vi "IVIS FRET_Compute Ratios.vi"(9 "g":dbl=1.0 min=0.0, 11 "Frame Image Components":T3) -> (1 "Frame Image Parameters":T2, 2 "Frame Image Intensities":T1, 3 "Frame Image Outputs":T5)   [LabVIEW 2021]
uses:
  IVIS FRET_Frame Image Outputs.ctl
  IVIS FRET_Frame Image Components Data.ctl
  Image/Image Point.ctl
  IVIS FRET_Frame Image Parameters.ctl
  IVIS FRET_Frame Image Intensities.ctl
  b41ef2ff-39d0-4c19-96d8-b3aa1b28ecf1.vi
  7645d199-fdb0-4455-8b8c-9fcb5e39c3d7.vi
  9ac8a814-4e7f-4100-867f-6759366377cb.vi
  41b5a819-f782-48c6-95c8-fb2ee3cdc111.vi
  b41ef2ff-39d0-4c19-96d8-b3aa1b28ecf1.vi/1ce800e1-bcd7-4855-83e2-66cab3687e54.vi
  7645d199-fdb0-4455-8b8c-9fcb5e39c3d7.vi/1ce800e1-bcd7-4855-83e2-66cab3687e54.vi
  9ac8a814-4e7f-4100-867f-6759366377cb.vi/1ce800e1-bcd7-4855-83e2-66cab3687e54.vi
  41b5a819-f782-48c6-95c8-fb2ee3cdc111.vi/1ce800e1-bcd7-4855-83e2-66cab3687e54.vi
  <vilib>/Analysis/NI_AALBase.lvlib
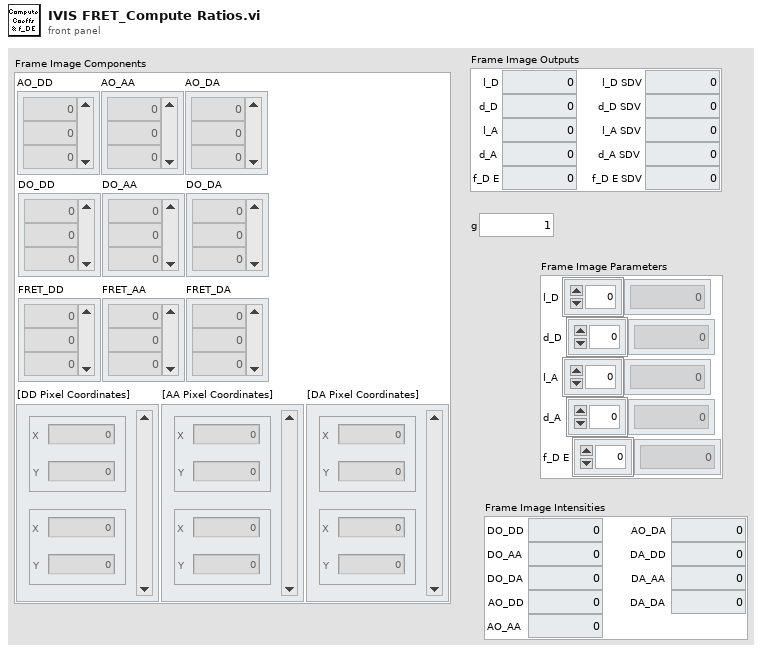
[diagram p1: front panel]
types:
  T1 = typedef "IVIS FRET_Frame Image Intensities.ctl" = cluster{"DO_DD":dbl, "DO_AA":dbl, "DO_DA":dbl, "AO_DD":dbl, "AO_AA":dbl, "AO_DA":dbl, "DA_DD":dbl, "DA_AA":dbl, "DA_DA":dbl}
  T2 = typedef "IVIS FRET_Frame Image Parameters.ctl" = cluster{"l_D":dbl[], "d_D":dbl[], "l_A":dbl[], "d_A":dbl[], "f_D E":dbl[]}
  T3 = typedef "IVIS FRET_Frame Image Components Data.ctl" = cluster{"AO_DD":sgl[], "AO_AA":sgl[], "AO_DA":sgl[], "DO_DA":sgl[], "DO_AA":sgl[], "DO_DD":sgl[], "FRET_DA":sgl[], "FRET_AA":sgl[], "FRET_DD":sgl[], "[DD Pixel Coordinates]":T4[], "[AA Pixel Coordinates]":T4[], "[DA Pixel Coordinates]":T4[]}
  T4 = typedef "Image Point.ctl" = cluster{"X":i32, "Y":i32}
  T5 = typedef "IVIS FRET_Frame Image Outputs.ctl" = cluster{"l_D":dbl, "l_D SDV":dbl, "d_D":dbl, "d_D SDV":dbl, "l_A":dbl, "l_A SDV":dbl, "d_A":dbl, "d_A SDV":dbl, "f_D E":dbl, "f_D E SDV":dbl}
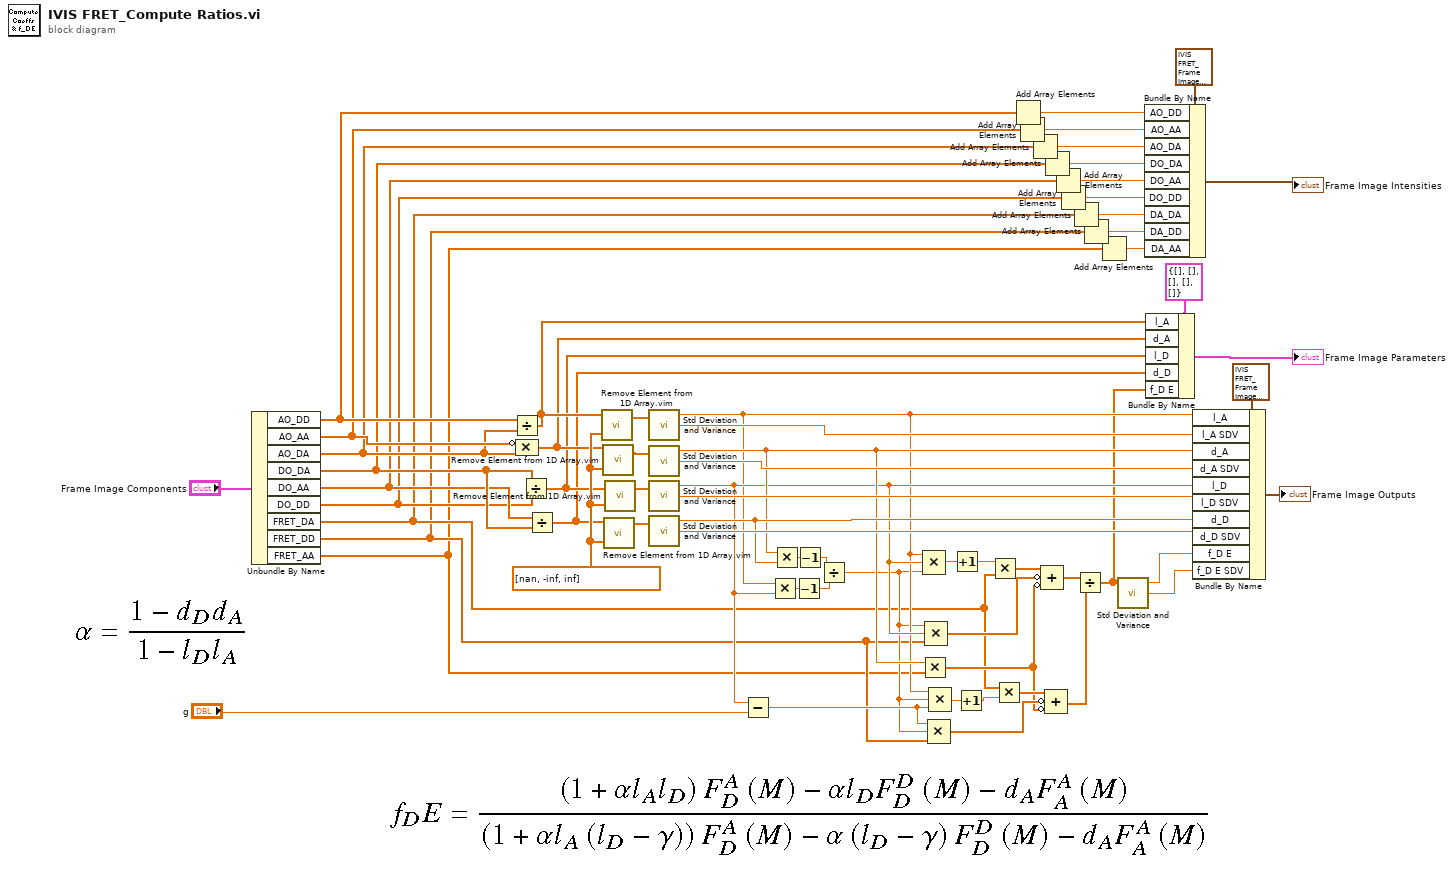
[diagram p0: block diagram]
diagram:
  w28 = dbl[] [nan, -inf, inf] ("Element(s) to Remove")
  n1 = Unbundle By Name("Frame Image Components") -> ("AO_DD"=w18:sgl[], "AO_AA"=w17:sgl[], "AO_DA"=w16:sgl[], "DO_DA"=w15:sgl[], "DO_AA"=w14:sgl[], "DO_DD"=w13:sgl[], "FRET_DA"=w12:sgl[], "FRET_DD"=w11:sgl[], "FRET_AA"=w10:sgl[])
  n2 = Divide(x=w18, y=w16) -> (x/y=w25:sgl[])
  n3 = Compound Arithmetic op=MULTIPLY(invert w17, w16) -> (w24:sgl[])
  n4 = Divide(x=w15, y=w13) -> (x/y=w23:sgl[])
  n5 = Divide(x=w14, y=w15) -> (x/y=w22:sgl[])
  n6 = call "Remove Element from 1D Array.vim"("Element(s) to Remove"=w28, "Input Array"=w25) -> ("Output Array"=w32:sgl[])  [unwired: 1 out]
  n7 = call "Remove Element from 1D Array.vim"("Element(s) to Remove"=w28, "Input Array"=w24) -> ("Output Array"=w29:sgl[])  [unwired: 1 out]
  n8 = call "Remove Element from 1D Array.vim"("Element(s) to Remove"=w28, "Input Array"=w22) -> ("Output Array"=w30:sgl[])  [unwired: 1 out]
  n9 = call "Remove Element from 1D Array.vim"("Element(s) to Remove"=w28, "Input Array"=w23) -> ("Output Array"=w31:sgl[])  [unwired: 1 out]
  n10 = call <vilib>:"Std Deviation and Variance.vi"("X"=w32) -> ("mean"=w44:dbl, "standard deviation"=w59:dbl)  [unwired: 1 in, 1 out]
  n11 = call <vilib>:"Std Deviation and Variance.vi"("X"=w29) -> ("mean"=w47:dbl, "standard deviation"=w57:dbl)  [unwired: 1 in, 1 out]
  n12 = call <vilib>:"Std Deviation and Variance.vi"("X"=w31) -> ("mean"=w46:dbl, "standard deviation"=w61:dbl)  [unwired: 1 in, 1 out]
  n13 = call <vilib>:"Std Deviation and Variance.vi"("X"=w30) -> ("mean"=w56:dbl, "standard deviation"=w58:dbl)  [unwired: 1 in, 1 out]
  n14 = Subtract(x=w46, y="g") -> (x-y=w40:dbl)
  n15 = Multiply(x=w44, y=w46) -> (x*y=w54:dbl)
  n16 = Multiply(x=w47, y=w56) -> (x*y=w55:dbl)
  n17 = Decrement(x=w54) -> (x-1=w52:dbl)
  n18 = Decrement(x=w55) -> (x-1=w53:dbl)
  n19 = Divide(x=w53, y=w52) -> (x/y=w39:dbl)
  n20 = Multiply(x=w47, y=w10) -> (x*y=w37:dbl[])
  n21 = Compound Arithmetic op=MULTIPLY(w44, w46, w39) -> (w51:dbl)
  n22 = Compound Arithmetic op=MULTIPLY(w39, w46, w11) -> (w48:dbl[])
  n23 = Compound Arithmetic op=MULTIPLY(w40, w39, w11) -> (w38:dbl[])
  n24 = Compound Arithmetic op=MULTIPLY(w44, w39, w40) -> (w43:dbl)
  n25 = Increment(x=w51) -> (x+1=w50:dbl)
  n26 = Increment(x=w43) -> (x+1=w42:dbl)
  n27 = Multiply(x=w50, y=w12) -> (x*y=w49:dbl[])
  n28 = Multiply(x=w12, y=w42) -> (x*y=w41:dbl[])
  n29 = Add Array Elements(numeric array=w18) -> (sum=w9:sgl)
  n30 = Add Array Elements(numeric array=w17) -> (sum=w8:sgl)
  n31 = Add Array Elements(numeric array=w16) -> (sum=w7:sgl)
  n32 = Compound Arithmetic op=ADD(w49, invert w48, invert w37) -> (w36:dbl[])
  n33 = Add Array Elements(numeric array=w15) -> (sum=w6:sgl)
  n34 = Compound Arithmetic op=ADD(w41, invert w38, invert w37) -> (w35:dbl[])
  n35 = Add Array Elements(numeric array=w14) -> (sum=w5:sgl)
  n36 = Add Array Elements(numeric array=w13) -> (sum=w4:sgl)
  n37 = Add Array Elements(numeric array=w12) -> (sum=w3:sgl)
  n38 = Divide(x=w36, y=w35) -> (x/y=w21:dbl[])
  n39 = Add Array Elements(numeric array=w11) -> (sum=w2:sgl)
  n40 = Add Array Elements(numeric array=w10) -> (sum=w1:sgl)
  n41 = call <vilib>:"Std Deviation and Variance.vi"("X"=w21) -> ("mean"=w34:dbl, "standard deviation"=w33:dbl)  [unwired: 1 in, 1 out]
  n42 = Bundle By Name(cluster=T1 {"DO_DD"=0.0, "DO_AA"=0.0, "DO_DA"=0.0, "AO_DD"=0.0, "AO_AA"=0.0, "AO_DA"=0.0, "DA_DD"=0.0, "DA_AA"=0.0, "DA_DA"=0.0} ("Frame Image Intensities"), "AO_DD"=w9, "AO_AA"=w8, "AO_DA"=w7, "DO_DA"=w6, "DO_AA"=w5, "DO_DD"=w4, "DA_DA"=w3, "DA_DD"=w2, "DA_AA"=w1) -> (→"Frame Image Intensities":T1)
  n43 = Bundle By Name(cluster=T2 {"l_D"=[], "d_D"=[], "l_A"=[], "d_A"=[], "f_D E"=[]} ("Frame Image Parameters"), "l_A"=w25, "d_A"=w24, "l_D"=w23, "d_D"=w22, "f_D E"=w21) -> (→"Frame Image Parameters":T2)
  n44 = Bundle By Name(cluster=T5 {"l_D"=0.0, "l_D SDV"=0.0, "d_D"=0.0, "d_D SDV"=0.0, "l_A"=0.0, "l_A SDV"=0.0, "d_A"=0.0, "d_A SDV"=0.0, "f_D E"=0.0, "f_D E SDV"=0.0} ("Frame Image Outputs"), "l_A"=w44, "l_A SDV"=w59, "d_A"=w47, "d_A SDV"=w57, "l_D"=w46, "l_D SDV"=w61, "d_D"=w56, "d_D SDV"=w58, "f_D E"=w34, "f_D E SDV"=w33) -> (→"Frame Image Outputs":T5)
